vi "Draw Graph.vi"(7 "History Graph State in":T1, 8 "error in (no error)":errorcluster, 9 "Scrollbar in":u64(c297), 10 "Live Button":bool) -> (0 "error out":errorcluster, 1 "Scrollbar out":u64, 2 "Waveform Graph":waveform(dbl)[](graph), 4 "Number of values in file":u64, 5 "History Graph State out":T1)   [LabVIEW 2018, in "History Graph.lvlib"]
uses:
  History Graph.lvlib
  Controls/History Graph State Cluster.ctl
panel:
  out "group/channel names":string[][](array[string])
  out "group names":string[](array[string])
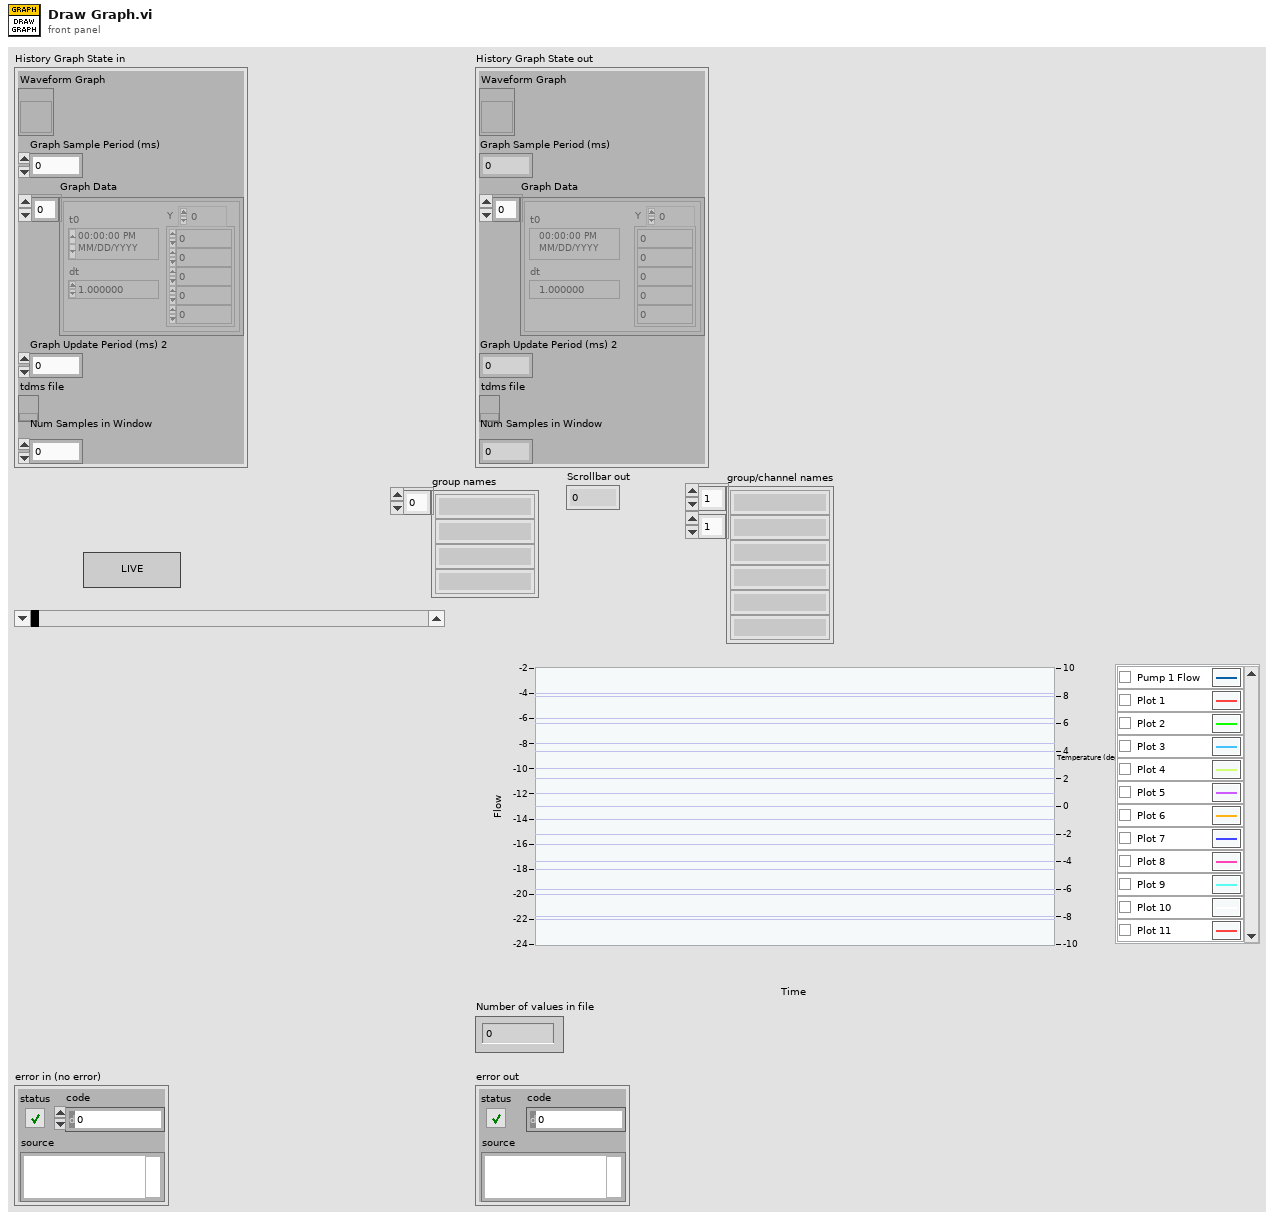
[diagram p1: front panel]
types:
  T1 = typedef "History Graph.lvlib/History Graph State Cluster.ctl" = cluster{"Waveform Graph":refnum<vi>, "Graph Sample Period (ms)":i32, "Graph Data":waveform(dbl)[], "Graph Update Period (ms) 2":i32, "tdms file":refnum<k34>, "Num Samples in Window":i64}
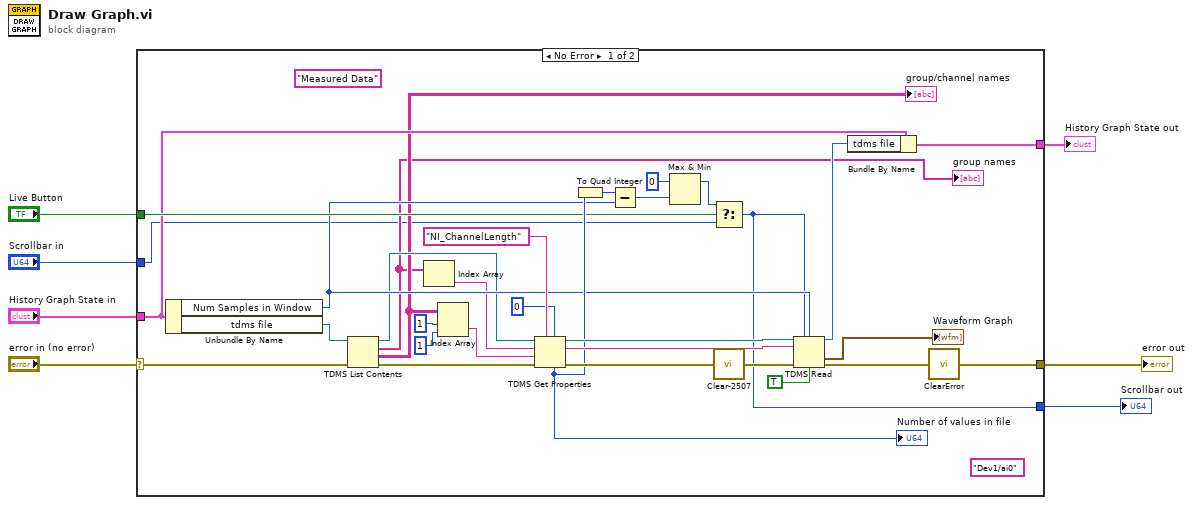
[diagram p0: block diagram]
diagram:
  n1 = case shown="No Error" "error in (no error)" {
    selector: "error in (no error)" -> [w18 w41]
    tunnel: [w26 w41] -> w5
    tunnel: "History Graph State in" -> [w23 w42]
    tunnel: [w24 w42] -> w7
    tunnel: "Live Button" -> [w29 _]
    tunnel: [w10 w40] -> w2
    tunnel: "Scrollbar in" -> [w9 w40]
    frame No Error {
      (unwired) "Measured Data" ("channel name(s) in")
      (unwired) "Dev1/ai0" ("channel name")
      n2 = Unbundle By Name(w23) -> ("Num Samples in Window"=w25:i64, "tdms file"=w20:refnum<k34>)
      n3 = TDMS List Contents(4:w18, 7:w20) -> (0:w17:errorcluster, 1:w16:string[][], 2:w13:string[], 3:w19:refnum<k34>)  [unwired: 1 in]
      "group names" <- w13
      "group/channel names" <- w16
      n4 = Index Array(array=w13) -> (element=w12:string)  [unwired: 1 in]
      n5 = Index Array(array=w16, index (row)=1, index (col)=1 ("disabled index (col)")) -> (element=w8:string)
      n6 = TDMS Get Properties(5:u64 0, 7:"NI_ChannelLength" ("channel name(s) in"), 8:w17, 9:w8, 10:w12, 11:w19) -> (0:w35:errorcluster, 2:w36:string, 3:w37:refnum<k34>, 4:w33:u64)  [unwired: 2 out]
      "Number of values in file" <- w33
      n7 = To Quad Integer(1:w33) -> (0:w11:i64)
      n8 = Subtract(x=w11, y=w25) -> (x-y=w31:i64)
      n9 = Max & Min(x=i64 0, y=w31) -> (max(x,y)=w30:i64)  [unwired: 1 out]
      n10 = Select(t=w30, s=w29, f=w9) -> (s? t:f=w10:u64)
      n11 = call <vilib>:"Clear-2507.vi"("error in (no error)"=w35) -> ("error out"=w34:errorcluster)
      n12 = TDMS Read(0:w37, 1:w10, 2:w25, 5:w36, 11:w34, 13:TRUE ("return channels in file order? (F)")) -> (4:w22:refnum<k34>, 10:→"Waveform Graph":waveform(dbl)[], 15:w28:errorcluster)  [unwired: 2 in, 3 out]
      n13 = Bundle By Name(cluster=w23, "tdms file"=w22) -> (w24:T1)
      n14 = call <vilib>:"ClearError.vi"("error in (no error)"=w28) -> ("error out"=w26:errorcluster)
    }
    frame Error {
    }
  }
  "History Graph State out" <- w7
  "error out" <- w5
  "Scrollbar out" <- w2
